vi "Map Channels In Engine.vi"(8 "error in (no error)":errorcluster, 9 "channels":refnum<class "TBM channel.lvclass">[](array[class]), 10 "instance id":string, 11 "Engine DVR":refnum<data-value>) -> (0 "error out":errorcluster)   [LabVIEW 2013, in "control module editor.lvclass"]
uses:
  control module editor.lvclass
  Configuration Editor/Classes/Engine Parent/Engine Parent Editor Node.lvclass
  <vilib>/NI/Tag Bus Module Framework/channel/TBM channel.lvclass
  <vilib>/NI/Module Execution Interface/Engine Configuration/engine configuration.lvclass
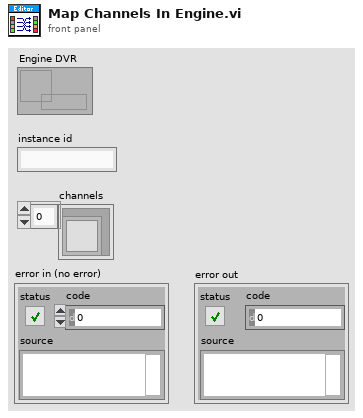
[diagram p1: front panel]
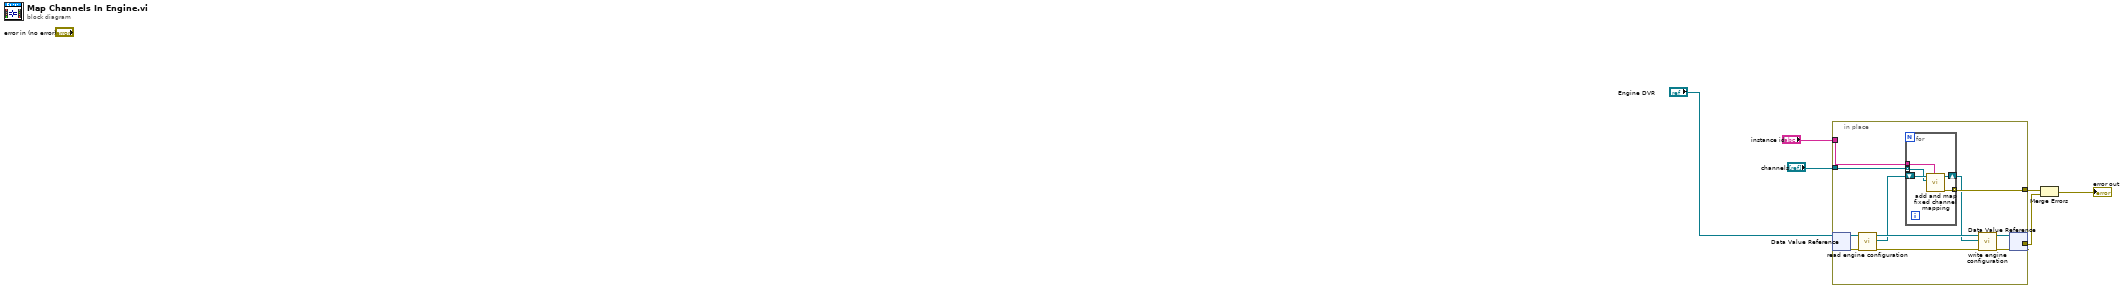
[diagram p0: block diagram]
diagram:
  n1 = in-place {
    in-place-border: [w17] -> w1
    in-place-border: [w13] -> w2
    in-place-border: "channels" -> [w9]
    in-place-border: "instance id" -> [w7]
    n2 = in-place-dvr #1("Engine DVR") -> (w15:refnum<class "Engine Parent Editor Node.lvclass">, w16:errorcluster)
    n3 = call "read engine configuration.vi"("error in"=w16, "Engine Parent Editor Node in"=w15) -> ("error out"=w12:errorcluster, "engine configuration"=w10:refnum<class "engine configuration.lvclass">, "Engine Parent Editor Node out"=w11:refnum<class "Engine Parent Editor Node.lvclass">)  [unwired: 7 in]
    n4 = for {
      tunnel: [w22] -> w17 mode=indexing
      shift-right: [w20] -> w8
      shift-left: w10 -> [w21]
      tunnel: w9 -> [w19] mode=indexing
      tunnel: w7 -> [w18]
      n5 = call <vilib>:"add and map fixed channel mapping.vi"("module instance"=w18, "fixed channel"=w19, "engine configuration in"=w21) -> ("error out"=w22:errorcluster, "engine configuration out"=w20:refnum<class "engine configuration.lvclass">)  [unwired: 7 in]
    }
    n6 = call "write engine configuration.vi"("error in"=w12, "engine configuration"=w8, "Engine Parent Editor Node in"=w11) -> ("error out"=w13:errorcluster, "Engine Parent Editor Node out"=w14:refnum<class "Engine Parent Editor Node.lvclass">)  [unwired: 7 in]
    n7 = in-place-dvr #1(w14) -> ()  [unwired: 2 out]
  }
  n8 = Merge Errors(w1, w2) -> (→"error out":errorcluster)
